vi "Result.Test Result to CSV.vi"(6 "SummaryOnly":bool, 7 "Exclude Header CSV":bool, 8 "error in":errorcluster, 9 "Test Result":T1={"#attributes"={"Version"="MTE_1.0.0"}, "Station"={"Name"="", "PN"="", "SN"="", "Rev"="", "PC Name"="", "Location"="", "HW_Config"={"HW_Item"=[]}, "SW_Config"={"SW_Item"=[]}}, "Test Run"={"Operator"="", "Start Time"=timestamp(0 s since 1904-01-01), "Duration(s)"=0.0, "Mode"="", "Comment"="", "ProcessStep"=""}, "Test Sequence"={"Name"="", "Config"={"Config_Item"=[]}}, "UUTs"={"UUT"=[]}} {"UUTs"."UUT"."Measurements"."Measurement"."Status" items=["LOG", "PASS", "FAIL", "ERROR"]}, 10 "File Name":string, 11 "Dir":path) -> (0 "error out":errorcluster, 3 "File Out":path)   [LabVIEW 2018]
uses:
  Result XML/TestResult.FullResultData.ctl
  Result XML/TestResult.Station Info.ctl
  Result XML/TestResult.HW Item.ctl
  Result XML/TestResult.SW Item.ctl
  Result XML/TestResult.Test Run Info.ctl
  Result XML/TestResult.Test Info.ctl
  Result XML/TestResult.UUT Result.ctl
  Result XML/TestResult.Symptom.ctl
  Result XML/TestResult.Symptom.State.ctl
  Result.Measurement Item.ctl
  Result.Measurement and Attribute Item Status.ctl
  Result XML/TestResult.UUTInfo.ctl
  <vilib>/KATE/Files/File Utils.lvlib
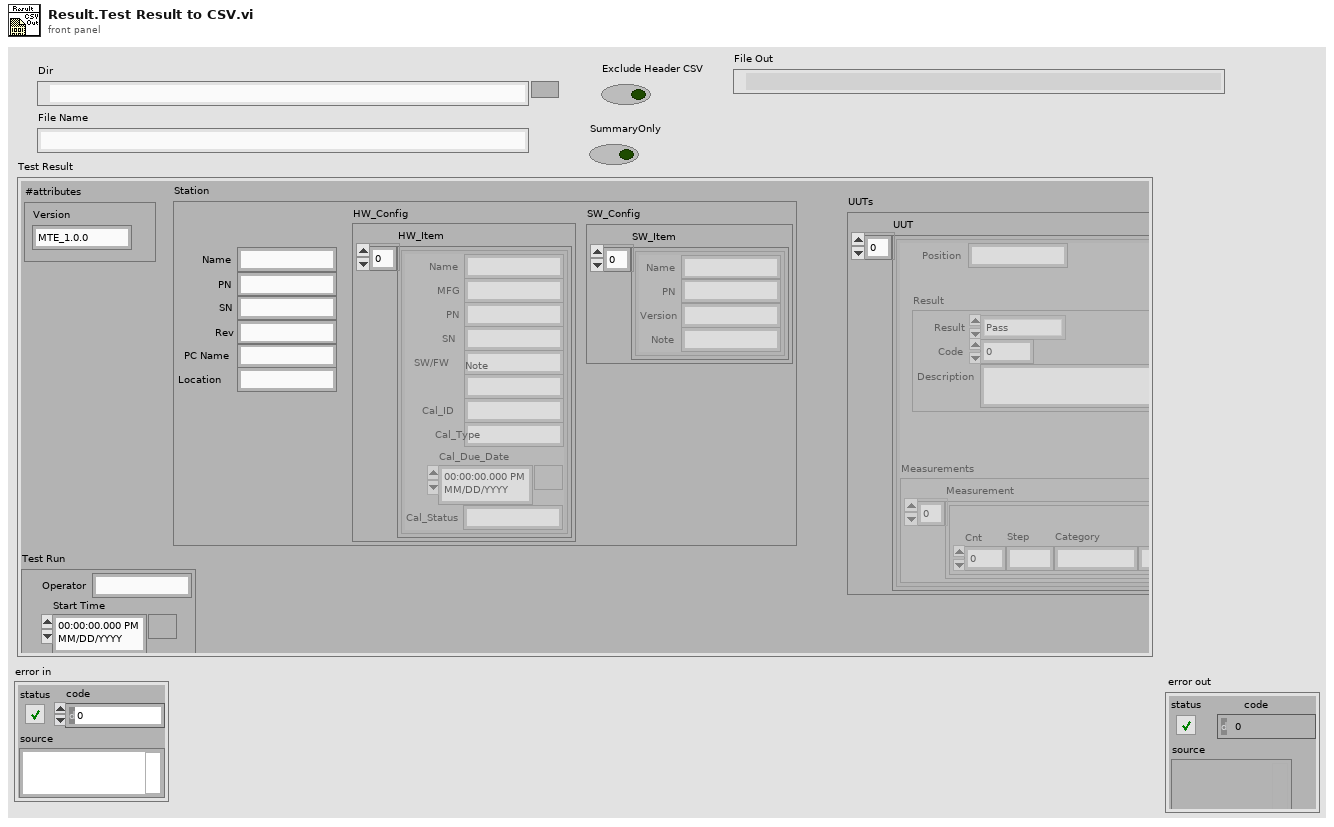
[diagram p1: front panel]
types:
  T1 = typedef "TestResult.FullResultData.ctl" = cluster{"#attributes":cluster{"Version":string}, "Station":T2, "Test Run":T5, "Test Sequence":T6, "UUTs":cluster{"UUT":T7[]}}
  T2 = typedef "TestResult.Station Info.ctl" = cluster{"Name":string, "PN":string, "SN":string, "Rev":string, "PC Name":string, "Location":string, "HW_Config":cluster{"HW_Item":T3[]}, "SW_Config":cluster{"SW_Item":T4[]}}
  T3 = typedef "TestResult.HW Item.ctl" = cluster{"Name":string, "MFG":string, "PN":string, "SN":string, "SW/FW":string, "Note":string, "Cal_ID":string, "Cal_Type":string, "Cal_Due_Date":timestamp, "Cal_Status":string}
  T4 = typedef "TestResult.SW Item.ctl" = cluster{"Name":string, "PN":string, "Version":string, "Note":string}
  T5 = typedef "TestResult.Test Run Info.ctl" = cluster{"Operator":string, "Start Time":timestamp, "Duration(s)":dbl, "Mode":string, "Comment":string, "ProcessStep":string}
  T6 = typedef "TestResult.Test Info.ctl" = cluster{"Name":string, "Config":cluster{"Config_Item":cluster{"Name":string, "Value":string}[]}}
  T7 = typedef "TestResult.UUT Result.ctl" = cluster{"Position":string, "Result":T8, "Measurements":cluster{"Measurement":T10[]}, "UUTInfo":T12}
  T8 = typedef "TestResult.Symptom.ctl" = cluster{"Result":T9, "Code":i32, "Description":string}
  T9 = typedef "TestResult.Symptom.State.ctl" = enum16{"Pass", "Fail", "Error", "Aborted", "Completed", "Logged"}
  T10 = typedef "Result.Measurement Item.ctl" = cluster{"Cnt":i32, "Step":string, "Category":string, "Name":string, "Value":string, "Units":string, "LimType":string, "LL":string, "UL":string, "Status":T11, "Code":i32, "Desc":string, "Time":timestamp}
  T11 = typedef "Result.Measurement and Attribute Item Status.ctl" = i32
  T12 = typedef "TestResult.UUTInfo.ctl" = cluster{"Product":string, "Desc":string, "PN":string, "SN":string, "Lot":string, "DateCode":string, "AltID":string, "Revision":string, "Properties":cluster{"Property":cluster{"Name":string, "Value":string}[]}}
  T13 = enum16{"open", "replace", "create", "open or create", "replace or create", "replace or create with confirmation"}
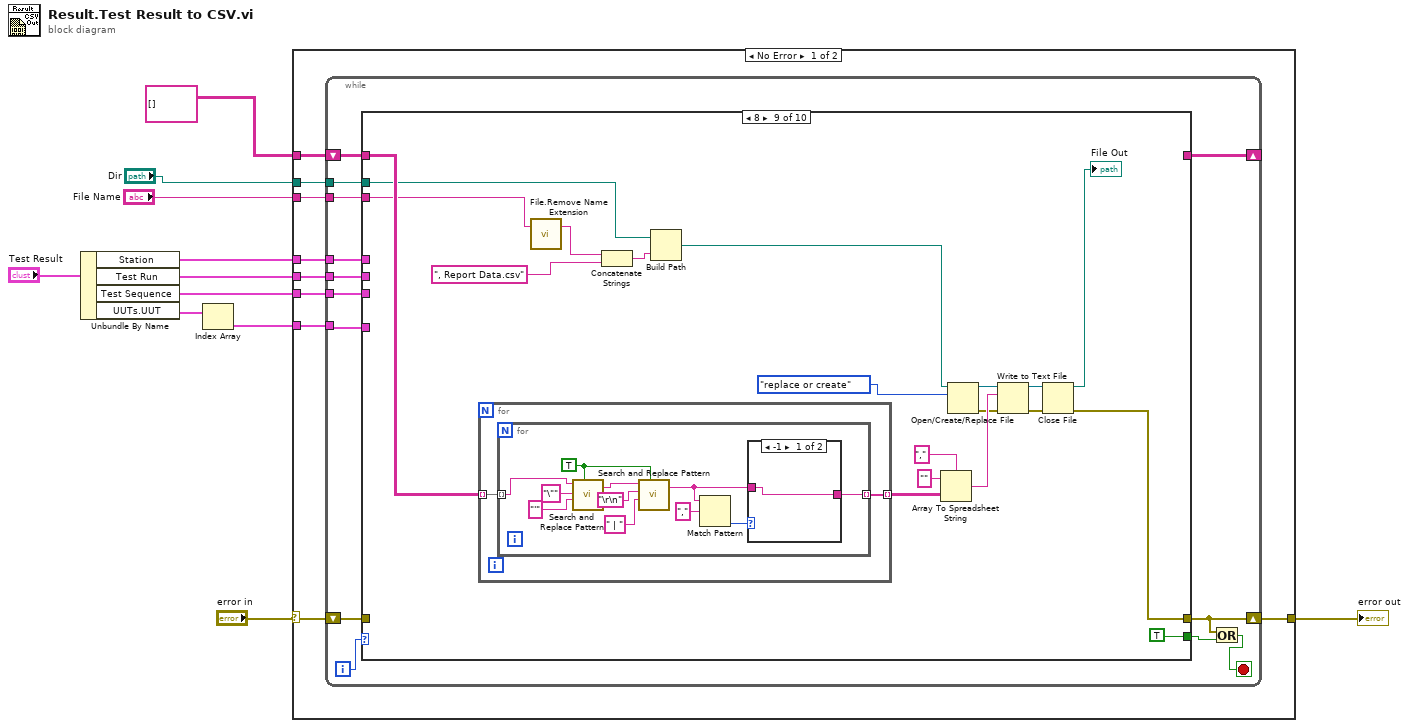
[diagram p0: block diagram]
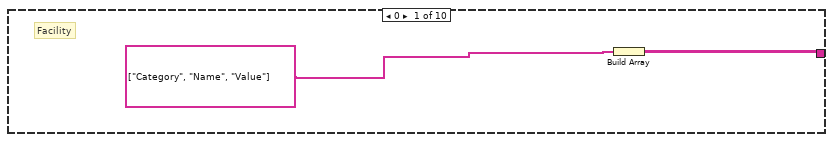
[diagram p2: hidden frame]
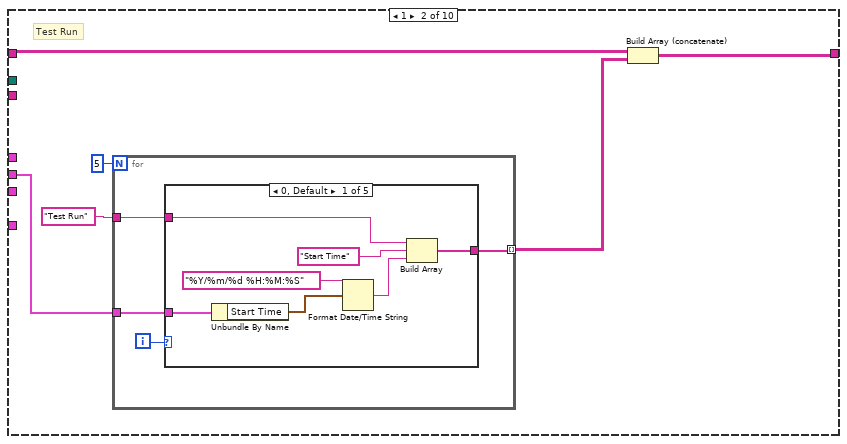
[diagram p3: hidden frame]
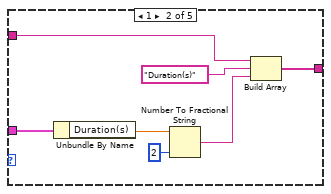
[diagram p4: hidden frame]
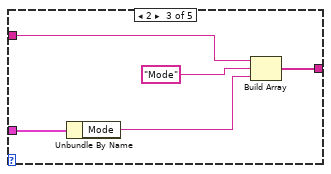
[diagram p5: hidden frame]
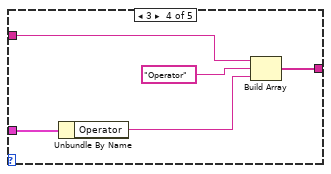
[diagram p6: hidden frame]
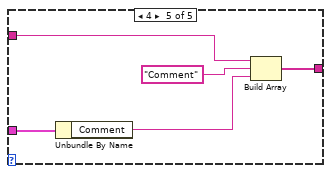
[diagram p7: hidden frame]
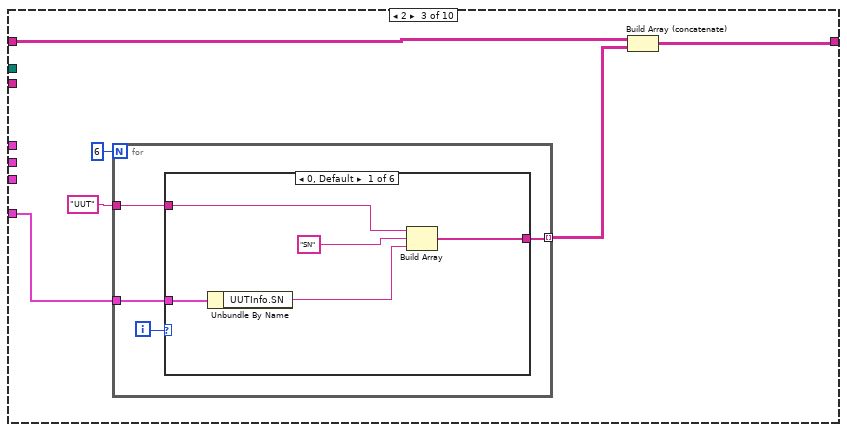
[diagram p8: hidden frame]
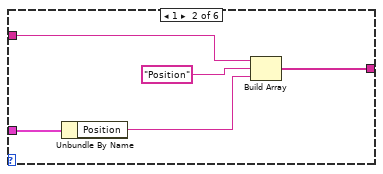
[diagram p9: hidden frame]
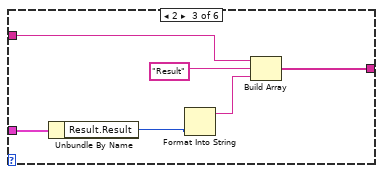
[diagram p10: hidden frame]
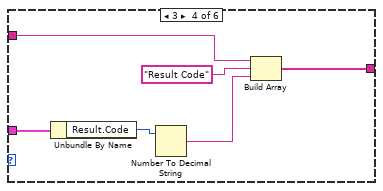
[diagram p11: hidden frame]
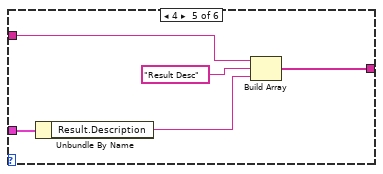
[diagram p12: hidden frame]
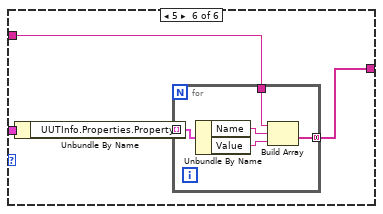
[diagram p13: hidden frame]
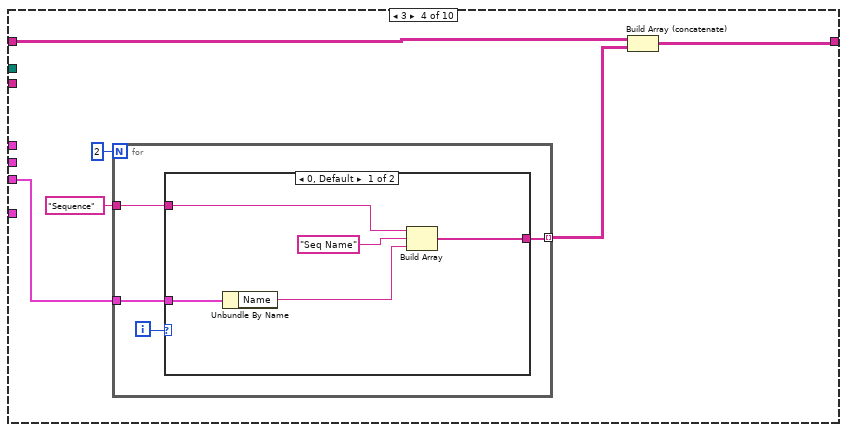
[diagram p14: hidden frame]
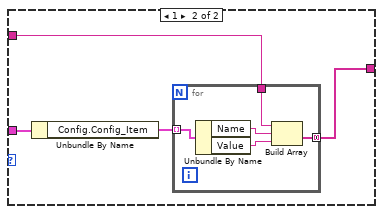
[diagram p15: hidden frame]
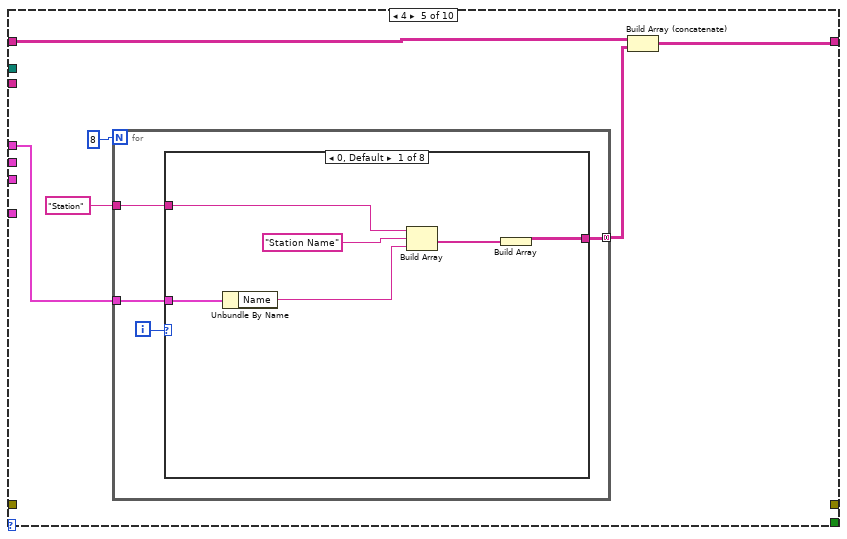
[diagram p16: hidden frame]
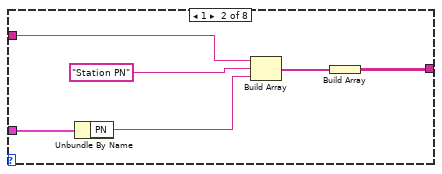
[diagram p17: hidden frame]
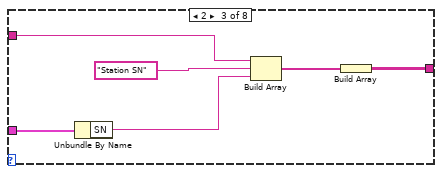
[diagram p18: hidden frame]
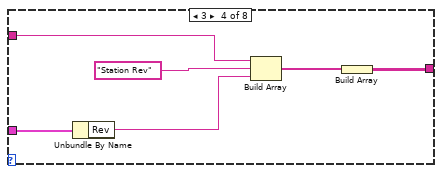
[diagram p19: hidden frame]
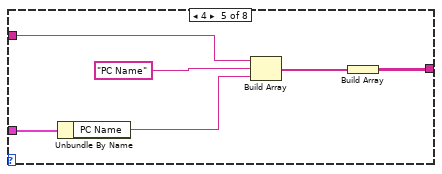
[diagram p20: hidden frame]
diagram:
  n1 = Unbundle By Name("Test Result") -> ("Station"=w6:T2, "Test Run"=w5:T5, "Test Sequence"=w4:T6, "UUTs.UUT"=w8:T7[])
  n2 = Index Array(array=w8) -> (element=w7:T7)  [unwired: 1 in]
  n3 = case shown="No Error" "error in" {
    selector: "error in" -> [w19 w492]
    tunnel: [w20 w492] -> w11
    tunnel: w7 -> [w18 _]
    tunnel: w6 -> [w17 _]
    tunnel: w5 -> [w16 _]
    tunnel: w4 -> [w15 _]
    tunnel: "File Name" -> [w14 _]
    tunnel: "Dir" -> [w13 _]
    tunnel: string[][] [] -> [w12 _]
    frame No Error {
      n4 = while {
        shift-right: [w23] -> w20
        shift-left: w19 -> [w33]
        shift-right: [w26] -> _
        shift-left: w12 -> [w32]
        tunnel: w18 -> [w29]
        tunnel: w17 -> [w28]
        tunnel: w16 -> [w30]
        tunnel: w15 -> [w27]
        tunnel: w14 -> [w25]
        tunnel: w13 -> [w24]
        i -> [w31]
        stop <- w21 stop-if-true
        n5 = case shown="8" w31 {
          tunnel: [_ _ _ _ _ w216 _ _ w455 w490] -> w23
          tunnel: w33 -> [_ _ _ _ _ _ _ _ _ w490]
          tunnel: w32 -> [_ w36 w77 w123 w148 w217 _ w429 w462 _]
          tunnel: [w35 w37 w75 w121 w145 _ w260 w430 _ _] -> w26
          tunnel: w30 -> [_ w38 _ _ _ _ w255 _ _ _]
          tunnel: w29 -> [_ _ w76 _ _ _ w258 w432 _ _]
          tunnel: w28 -> [_ _ _ _ w147 _ w254 _ _ _]
          tunnel: w27 -> [_ _ _ w122 _ _ w253 _ _ _]
          tunnel: [_ _ _ _ _ "SummaryOnly" _ _ TRUE TRUE] -> w22
          tunnel: w25 -> [_ _ _ _ _ w227 _ _ w458 _]
          tunnel: w24 -> [_ _ _ _ _ w224 _ _ w457 _]
          frame 0 {
            # "Facility"
            n6 = Build Array(string[] ["Category", "Name", "Value"]) -> (w35:string[][])
          }
          frame 1 {
            # "Test Run"
            n7 = for {
              N: 5 -> [_]
              tunnel: w38 -> [w45]
              tunnel: [w43] -> w39 mode=indexing
              tunnel: "Test Run" -> [w42]
              i -> [w44]
              n8 = case shown="0, Default" w44 {
                tunnel: w45 -> [w51 w59 w64 w69 w74]
                tunnel: [w47 w57 w62 w67 w72] -> w43
                tunnel: w42 -> [w46 w56 w61 w66 w71]
                frame 0, Default {
                  n9 = Unbundle By Name(w51) -> ("Start Time"=w48:timestamp)
                  n10 = Format Date/Time String(time format string (%c)="%Y/%m/%d %H:%M:%S", seconds (now)=w48) -> (date/time string=w49:string)  [unwired: 1 in]
                  n11 = Build Array(w46, "Start Time", w49) -> (w47:string[])
                }
                frame 1 {
                  n12 = Unbundle By Name(w59) -> ("Duration(s)"=w55:dbl)
                  n13 = Number To Fractional String(number=w55, precision (6)=i16 2) -> (F-format string=w53:string)  [unwired: 2 in]
                  n14 = Build Array(w56, "Duration(s)", w53) -> (w57:string[])
                }
                frame 2 {
                  n15 = Unbundle By Name(w64) -> ("Mode"=w60:string)
                  n16 = Build Array(w61, "Mode", w60) -> (w62:string[])
                }
                frame 3 {
                  n17 = Unbundle By Name(w69) -> ("Operator"=w65:string)
                  n18 = Build Array(w66, "Operator", w65) -> (w67:string[])
                }
                frame 4 {
                  n19 = Unbundle By Name(w74) -> ("Comment"=w70:string)
                  n20 = Build Array(w71, "Comment", w70) -> (w72:string[])
                }
              }
            }
            n21 = Build Array (concatenate)(w36, w39) -> (w37:string[][])
          }
          frame 2 {
            n22 = for {
              N: 6 -> [_]
              tunnel: w76 -> [w84]
              tunnel: [w82] -> w78 mode=indexing
              tunnel: "UUT" -> [w81]
              i -> [w83]
              n23 = case shown="0, Default" w83 {
                tunnel: w84 -> [w89 w94 w100 w106 w111 w115]
                tunnel: [w87 w92 w99 w104 w109 w112] -> w82
                tunnel: w81 -> [w86 w91 w98 w103 w108 w113]
                frame 0, Default {
                  n24 = Unbundle By Name(w89) -> ("UUTInfo.SN"=w85:string)
                  n25 = Build Array(w86, "SN", w85) -> (w87:string[])
                }
                frame 1 {
                  n26 = Unbundle By Name(w94) -> ("Position"=w90:string)
                  n27 = Build Array(w91, "Position", w90) -> (w92:string[])
                }
                frame 2 {
                  n28 = Unbundle By Name(w100) -> ("Result.Result"=w96:T9)
                  n29 = Format Into String(w96) -> (resulting string=w95:string)  [unwired: 3 in, 1 out]
                  n30 = Build Array(w98, "Result", w95) -> (w99:string[])
                }
                frame 3 {
                  n31 = Unbundle By Name(w106) -> ("Result.Code"=w102:i32)
                  n32 = Number To Decimal String(number=w102) -> (decimal integer string=w101:string)  [unwired: 1 in]
                  n33 = Build Array(w103, "Result Code", w101) -> (w104:string[])
                }
                frame 4 {
                  n34 = Unbundle By Name(w111) -> ("Result.Description"=w107:string)
                  n35 = Build Array(w108, "Result Desc", w107) -> (w109:string[])
                }
                frame 5 {
                  n36 = Unbundle By Name(w115) -> ("UUTInfo.Properties.Property"=w114:cluster{"Name":string, "Value":string}[])
                  n37 = for {
                    tunnel: w114 -> [w120] mode=indexing
                    tunnel: [w117] -> w112 mode=concatenating
                    tunnel: w113 -> [w116]
                    n38 = Unbundle By Name(w120) -> ("Name"=w119:string, "Value"=w118:string)
                    n39 = Build Array(w116, w119, w118) -> (w117:string[])
                  }
                }
              }
            }
            n40 = Build Array (concatenate)(w77, w78) -> (w75:string[][])
          }
          frame 3 {
            n41 = for {
              N: 2 -> [_]
              tunnel: w122 -> [w130]
              tunnel: [w128] -> w124 mode=indexing
              tunnel: "Sequence" -> [w127]
              i -> [w129]
              n42 = case shown="0, Default" w129 {
                tunnel: w130 -> [w135 w139]
                tunnel: [w133 w136] -> w128
                tunnel: w127 -> [w132 w137]
                frame 0, Default {
                  n43 = Unbundle By Name(w135) -> ("Name"=w131:string)
                  n44 = Build Array(w132, "Seq Name", w131) -> (w133:string[])
                }
                frame 1 {
                  n45 = Unbundle By Name(w139) -> ("Config.Config_Item"=w138:cluster{"Name":string, "Value":string}[])
                  n46 = for {
                    tunnel: w138 -> [w144] mode=indexing
                    tunnel: [w141] -> w136 mode=concatenating
                    tunnel: w137 -> [w140]
                    n47 = Unbundle By Name(w144) -> ("Name"=w143:string, "Value"=w142:string)
                    n48 = Build Array(w140, w143, w142) -> (w141:string[])
                  }
                }
              }
            }
            n49 = Build Array (concatenate)(w123, w124) -> (w121:string[][])
          }
          frame 4 {
            n50 = for {
              N: 8 -> [_]
              tunnel: w147 -> [w154]
              tunnel: [w152] -> w146 mode=concatenating
              tunnel: "Station" -> [w151]
              i -> [w153]
              n51 = case shown="0, Default" w153 {
                tunnel: w154 -> [w160 w166 w172 w178 w184 w190 w196 w205]
                tunnel: [w155 w161 w167 w173 w179 w185 w193 w202] -> w152
                tunnel: w151 -> [w158 w164 w171 w177 w183 w189 _ _]
                frame 0, Default {
                  n52 = Unbundle By Name(w160) -> ("Name"=w157:string)
                  n53 = Build Array(w158, "Station Name", w157) -> (w156:string[])
                  n54 = Build Array(w156) -> (w155:string[][])
                }
                frame 1 {
                  n55 = Unbundle By Name(w166) -> ("PN"=w163:string)
                  n56 = Build Array(w164, "Station PN", w163) -> (w162:string[])
                  n57 = Build Array(w162) -> (w161:string[][])
                }
                frame 2 {
                  n58 = Unbundle By Name(w172) -> ("SN"=w169:string)
                  n59 = Build Array(w171, "Station SN", w169) -> (w168:string[])
                  n60 = Build Array(w168) -> (w167:string[][])
                }
                frame 3 {
                  n61 = Unbundle By Name(w178) -> ("Rev"=w175:string)
                  n62 = Build Array(w177, "Station Rev", w175) -> (w174:string[])
                  n63 = Build Array(w174) -> (w173:string[][])
                }
                frame 4 {
                  n64 = Unbundle By Name(w184) -> ("PC Name"=w181:string)
                  n65 = Build Array(w183, "PC Name", w181) -> (w180:string[])
                  n66 = Build Array(w180) -> (w179:string[][])
                }
                frame 5 {
                  n67 = Unbundle By Name(w190) -> ("Location"=w187:string)
                  n68 = Build Array(w189, "Station Location", w187) -> (w186:string[])
                  n69 = Build Array(w186) -> (w185:string[][])
                }
                frame 6 {
                  n70 = Unbundle By Name(w196) -> ("HW_Config.HW_Item"=w195:T3[])
                  n71 = for {
                    tunnel: w195 -> [w197] mode=indexing
                    tunnel: [w198] -> w192 mode=indexing
                    tunnel: "Equipment List" -> [w199]
                    n72 = call "Result.Equipment List Item to 1D Array.vi"("Eq Item"=w197, "Category"=w199) -> ("List"=w198:string[])  [unwired: 9 in]
                  }
                  n73 = Build Array (concatenate)(string[] ["Category", "Name", "PN", "SN", "SW/FW", "Cal ID", "Cal Type", "Cal Due", "Cal Status"], w192) -> (w193:string[][])
                }
                frame 7 {
                  n74 = Unbundle By Name(w205) -> ("SW_Config.SW_Item"=w204:T4[])
                  n75 = for {
                    tunnel: w204 -> [w212] mode=indexing
                    tunnel: [w206] -> w201 mode=indexing
                    tunnel: "SW List" -> [w207]
                    n76 = Unbundle By Name(w212) -> ("Name"=w208:string, "PN"=w209:string, "Version"=w210:string, "Note"=w211:string)
                    n77 = Build Array(w207, w208, w209, w210, w211) -> (w206:string[])
                  }
                  n78 = Build Array (concatenate)(string[] ["Category", "Name", "PN", "Version", "Note"], w201) -> (w202:string[][])
                }
              }
            }
            n79 = Build Array (concatenate)(w148, w146) -> (w145:string[][])
          }
          frame 5 {
            n80 = for {
              tunnel: w217 -> [w237] mode=indexing
              tunnel: [w236] -> w222 mode=indexing
              n81 = for {
                tunnel: w237 -> [w245] mode=indexing
                tunnel: [w248] -> w236 mode=indexing
                w243 = TRUE ("replace all? (F)")
                n82 = call <vilib>:"Search and Replace Pattern.vi"("string"=w245, "regular expression (\"\")"="\"", "replace string (\"\")"="'", "replace all? (F)"=w243) -> ("result string"=w244:string)  [unwired: 1 in, 1 out]
                n83 = call <vilib>:"Search and Replace Pattern.vi"("string"=w244, "regular expression (\"\")"="\n", "replace string (\"\")"=" | ", "replace all? (F)"=w243) -> ("result string"=w240:string)  [unwired: 1 in, 1 out]
                n84 = Match Pattern(string=w240, regular expression=",") -> (offset past match=w238:i32)  [unwired: 1 in, 3 out]
                n85 = case shown="-1" w238 {
                  tunnel: [w249 w251] -> w248
                  tunnel: w240 -> [w249 w250]
                  frame -1 {
                  }
                  frame 0, Default {
                    w252 = "\""
                    n86 = Concatenate Strings(w252, w250, w252) -> (w251:string)
                  }
                }
              }
            }
            n87 = call <vilib>:"File.Remove Name Extension.vi"("File Name"=w227) -> ("Name Less Ext"=w215:string)  [unwired: 1 in, 1 out]
            n88 = Concatenate Strings(w215, ", Report Header.csv" ("string")) -> (w225:string)
            n89 = Build Path(base path=w224, name or relative path=w225) -> (appended path=w218:path)
            n90 = Array To Spreadsheet String(delimiter (Tab)=",", array=w222, 3:"" ("format string")) -> (spreadsheet string=w223:string)
            n91 = case shown="False" "Exclude Header CSV" {
              tunnel: w223 -> [w235 _]
              tunnel: T13."replace or create" ("operation (0:open)") -> [w230 _]
              tunnel: w218 -> [w229 _]
              tunnel: [w228 _] -> w216
              frame False {
                n92 = Open/Create/Replace File(file path (use dialog)=w229, operation (0:open)=w230) -> (refnum out=w232:refnum<file>, error out=w233:errorcluster)  [unwired: 4 in, 1 out]
                n93 = Write to Text File(file (use dialog)=w232, text=w235, error in=w233) -> (refnum out=w231:refnum<file>, error out=w234:errorcluster)  [unwired: 1 in, 1 out]
                n94 = Close File(refnum=w231, error in=w234) -> (error out=w228:errorcluster)  [unwired: 1 out]
              }
              frame True {
              }
            }
          }
          frame 6 {
            # "SN\nPosition\nTime\nMode\nComment\nResult\nCode\nDesc\nDur\nOper"
            n95 = while {
              tunnel: w258 -> [w269]
              tunnel: [w267] -> w257 mode=indexing if=w263
              tunnel: string[] ["0", "0", "Header"] -> [w266]
              tunnel: w255 -> [w265]
              tunnel: w254 -> [w264]
              tunnel: w253 -> [w262]
              i -> [w268]
              stop <- w261 stop-if-true
              n96 = case shown="1" w268 {
                tunnel: w269 -> [w270 w275 _ _ _ _ w305 w311 w316 _ _ _ _ _ _ _ _ _ _ _ _ _ _]
                tunnel: [w273 w278 w282 w290 w295 w300 w307 w313 w318 w324 w329 w334 w344 w353 w362 w371 w380 w389 w398 w407 w416 w425 w427] -> w267
                tunnel: w266 -> [w271 w276 w280 w288 w293 w298 w306 w312 w317 w320 w327 w332 _ _ _ _ _ _ _ _ _ _ w427]
                tunnel: w265 -> [_ _ w281 w287 _ w297 _ _ _ w319 w326 _ _ _ _ _ _ _ _ _ _ _ _]
                tunnel: w264 -> [_ _ _ _ _ _ _ _ _ _ _ w331 w343 w352 w361 w370 w379 w388 w397 w406 w415 w424 _]
                tunnel: [_ _ _ _ _ _ _ _ _ _ _ _ w336 w345 w354 w363 w372 w381 w390 w399 w408 w417 TRUE] -> w261
                tunnel: w262 -> [_ _ _ _ w292 _ _ _ _ _ _ _ _ _ _ _ _ _ _ _ _ _ _]
                frame 0 {
                  n97 = Unbundle By Name(w270) -> ("UUTInfo.SN"=w272:string)
                  n98 = Build Array (concatenate)(w271, "SN", w272) -> (w273:string[])
                }
                frame 1 {
                  n99 = Unbundle By Name(w275) -> ("Position"=w277:string)
                  n100 = Build Array (concatenate)(w276, "Position", w277) -> (w278:string[])
                }
                frame 2 {
                  n101 = Unbundle By Name(w281) -> ("Start Time"=w283:timestamp)
                  n102 = Format Date/Time String(time format string (%c)="%Y/%m/%d %H:%M:%S", seconds (now)=w283) -> (date/time string=w284:string)  [unwired: 1 in]
                  n103 = Build Array (concatenate)(w280, "Start Time", w284) -> (w282:string[])
                }
                frame 3 {
                  n104 = Unbundle By Name(w287) -> ("Mode"=w289:string)
                  n105 = Build Array (concatenate)(w288, "Mode", w289) -> (w290:string[])
                }
                frame 4 {
                  n106 = Unbundle By Name(w292) -> ("Name"=w294:string)
                  n107 = Build Array (concatenate)(w293, "Sequence", w294) -> (w295:string[])
                }
                frame 5 {
                  n108 = Unbundle By Name(w297) -> ("Comment"=w299:string)
                  n109 = Build Array (concatenate)(w298, "Comment", w299) -> (w300:string[])
                }
                frame 6 {
                  n110 = Unbundle By Name(w305) -> ("Result.Result"=w303:T9)
                  n111 = Format Into String(w303) -> (resulting string=w302:string)  [unwired: 3 in, 1 out]
                  n112 = Build Array (concatenate)(w306, "Result", w302) -> (w307:string[])
                }
                frame 7 {
                  n113 = Unbundle By Name(w311) -> ("Result.Code"=w309:i32)
                  n114 = Format Into String(w309) -> (resulting string=w308:string)  [unwired: 3 in, 1 out]
                  n115 = Build Array (concatenate)(w312, "Result Code", w308) -> (w313:string[])
                }
                frame 8 {
                  n116 = Unbundle By Name(w316) -> ("Result.Description"=w314:string)
                  n117 = Build Array (concatenate)(w317, "Result Desc", w314) -> (w318:string[])
                }
                frame 9 {
                  n118 = Unbundle By Name(w319) -> ("Duration(s)"=w323:dbl)
                  n119 = Number To Fractional String(number=w323, precision (6)=i16 2) -> (F-format string=w321:string)  [unwired: 2 in]
                  n120 = Build Array (concatenate)(w320, "Duration(s)", w321) -> (w324:string[])
                }
                frame 10 {
                  n121 = Unbundle By Name(w326) -> ("Operator"=w328:string)
                  n122 = Build Array (concatenate)(w327, "Operator", w328) -> (w329:string[])
                }
                frame 11 {
                  n123 = Unbundle By Name(w331) -> ("Location"=w333:string)
                  n124 = Build Array (concatenate)(w332, "Location", w333) -> (w334:string[])
                }
                frame 12 {
                  n125 = Unbundle By Name(w343) -> ("SW_Config.SW_Item"=w342:T4[])
                  n126 = Index Array(array=w342, index=0) -> (element=w341:T4)
                  n127 = Unbundle By Name(w341) -> ("Name"=w339:string, "Version"=w340:string)
                  n128 = Build Array (concatenate)(string[] ["0", "0", "SW"], w339, w340) -> (w344:string[])
                  n129 = Empty String/Path?(string/path=w339) -> (empty?=w336:bool)
                }
                frame 13 {
                  n130 = Unbundle By Name(w352) -> ("SW_Config.SW_Item"=w351:T4[])
                  n131 = Index Array(array=w351, index=1) -> (element=w350:T4)
                  n132 = Unbundle By Name(w350) -> ("Name"=w348:string, "Version"=w349:string)
                  n133 = Build Array (concatenate)(string[] ["0", "0", "SW"], w348, w349) -> (w353:string[])
                  n134 = Empty String/Path?(string/path=w348) -> (empty?=w345:bool)
                }
                frame 14 {
                  n135 = Unbundle By Name(w361) -> ("SW_Config.SW_Item"=w360:T4[])
                  n136 = Index Array(array=w360, index=2) -> (element=w359:T4)
                  n137 = Unbundle By Name(w359) -> ("Name"=w357:string, "Version"=w358:string)
                  n138 = Build Array (concatenate)(string[] ["0", "0", "SW"], w357, w358) -> (w362:string[])
                  n139 = Empty String/Path?(string/path=w357) -> (empty?=w354:bool)
                }
                frame 15 {
                  n140 = Unbundle By Name(w370) -> ("SW_Config.SW_Item"=w369:T4[])
                  n141 = Index Array(array=w369, index=3) -> (element=w368:T4)
                  n142 = Unbundle By Name(w368) -> ("Name"=w366:string, "Version"=w367:string)
                  n143 = Build Array (concatenate)(string[] ["0", "0", "SW"], w366, w367) -> (w371:string[])
                  n144 = Empty String/Path?(string/path=w366) -> (empty?=w363:bool)
                }
                frame 16 {
                  n145 = Unbundle By Name(w379) -> ("SW_Config.SW_Item"=w378:T4[])
                  n146 = Index Array(array=w378, index=4) -> (element=w377:T4)
                  n147 = Unbundle By Name(w377) -> ("Name"=w375:string, "Version"=w376:string)
                  n148 = Build Array (concatenate)(string[] ["0", "0", "SW"], w375, w376) -> (w380:string[])
                  n149 = Empty String/Path?(string/path=w375) -> (empty?=w372:bool)
                }
                frame 17 {
                  n150 = Unbundle By Name(w388) -> ("SW_Config.SW_Item"=w387:T4[])
                  n151 = Index Array(array=w387, index=5) -> (element=w386:T4)
                  n152 = Unbundle By Name(w386) -> ("Name"=w384:string, "Version"=w385:string)
                  n153 = Build Array (concatenate)(string[] ["0", "0", "SW"], w384, w385) -> (w389:string[])
                  n154 = Empty String/Path?(string/path=w384) -> (empty?=w381:bool)
                }
                frame 18 {
                  n155 = Unbundle By Name(w397) -> ("SW_Config.SW_Item"=w396:T4[])
                  n156 = Index Array(array=w396, index=6) -> (element=w395:T4)
                  n157 = Unbundle By Name(w395) -> ("Name"=w393:string, "Version"=w394:string)
                  n158 = Build Array (concatenate)(string[] ["0", "0", "SW"], w393, w394) -> (w398:string[])
                  n159 = Empty String/Path?(string/path=w393) -> (empty?=w390:bool)
                }
                frame 19 {
                  n160 = Unbundle By Name(w406) -> ("SW_Config.SW_Item"=w405:T4[])
                  n161 = Index Array(array=w405, index=7) -> (element=w404:T4)
                  n162 = Unbundle By Name(w404) -> ("Name"=w402:string, "Version"=w403:string)
                  n163 = Build Array (concatenate)(string[] ["0", "0", "SW"], w402, w403) -> (w407:string[])
                  n164 = Empty String/Path?(string/path=w402) -> (empty?=w399:bool)
                }
                frame 20 {
                  n165 = Unbundle By Name(w415) -> ("SW_Config.SW_Item"=w414:T4[])
                  n166 = Index Array(array=w414, index=8) -> (element=w413:T4)
                  n167 = Unbundle By Name(w413) -> ("Name"=w411:string, "Version"=w412:string)
                  n168 = Build Array (concatenate)(string[] ["0", "0", "SW"], w411, w412) -> (w416:string[])
                  n169 = Empty String/Path?(string/path=w411) -> (empty?=w408:bool)
                }
                frame 21 {
                  n170 = Unbundle By Name(w424) -> ("SW_Config.SW_Item"=w423:T4[])
                  n171 = Index Array(array=w423, index=9) -> (element=w422:T4)
                  n172 = Unbundle By Name(w422) -> ("Name"=w420:string, "Version"=w421:string)
                  n173 = Build Array (concatenate)(string[] ["0", "0", "SW"], w420, w421) -> (w425:string[])
                  n174 = Empty String/Path?(string/path=w420) -> (empty?=w417:bool)
                }
                frame Default {
                }
              }
              n175 = Not(x=w261) -> (.not. x?=w263:bool)
            }
            n176 = Build Array (concatenate)(string[] ["Order", "Step", "Category", "Name", "Value", "Units", "LimType", "LL", "UL", "Result", "Result Code", "Result Desc"], w257) -> (w260:string[][])
          }
          frame 7 {
            (unwired) string[] ["Order", "Step", "Category", "Name", "Value", "Units", "LimType", "LL", "UL", "Result", "Result Code", "Result Desc"]
            n177 = Unbundle By Name(w432) -> ("Measurements.Measurement"=w428:T10[])
            n178 = for {
              tunnel: w428 -> [w449] mode=indexing
              tunnel: [w435] -> w431 mode=indexing
              n179 = Unbundle By Name(w449) -> ("Cnt"=w448:i32, "Step"=w446:string, "Category"=w445:string, "Name"=w444:string, "Value"=w443:string, "Units"=w442:string, "LimType"=w441:string, "LL"=w440:string, "UL"=w439:string, "Status"=w434:T11, "Code"=w438:i32, "Desc"=w436:string)
              n180 = case shown="3" w434 {
                tunnel: ["LOG" "PASS" "FAIL" "ERROR"] -> w433
                frame 0, Default {
                }
                frame 1 {
                }
                frame 2 {
                }
                frame 3 {
                }
              }
              n181 = Number To Decimal String(number=w448) -> (decimal integer string=w447:string)  [unwired: 1 in]
              n182 = Number To Decimal String(number=w438) -> (decimal integer string=w437:string)  [unwired: 1 in]
              n183 = Build Array(w447, w446, w445, w444, w443, w442, w441, w440, w439, w433, w437, w436) -> (w435:string[])
            }
            n184 = Build Array (concatenate)(w429, w431) -> (w430:string[][])
          }
          frame 8 {
            n185 = for {
              tunnel: w462 -> [w474] mode=indexing
              tunnel: [w473] -> w466 mode=indexing
              n186 = for {
                tunnel: w474 -> [w482] mode=indexing
                tunnel: [w485] -> w473 mode=indexing
                w480 = TRUE ("replace all? (F)")
                n187 = call <vilib>:"Search and Replace Pattern.vi"("string"=w482, "regular expression (\"\")"="\"", "replace string (\"\")"="'", "replace all? (F)"=w480) -> ("result string"=w481:string)  [unwired: 1 in, 1 out]
                n188 = call <vilib>:"Search and Replace Pattern.vi"("string"=w481, "regular expression (\"\")"="\r\n", "replace string (\"\")"=" | ", "replace all? (F)"=w480) -> ("result string"=w477:string)  [unwired: 1 in, 1 out]
                n189 = Match Pattern(string=w477, regular expression=",") -> (offset past match=w475:i32)  [unwired: 1 in, 3 out]
                n190 = case shown="-1" w475 {
                  tunnel: [w486 w488] -> w485
                  tunnel: w477 -> [w486 w487]
                  frame -1 {
                  }
                  frame 0, Default {
                    w489 = "\""
                    n191 = Concatenate Strings(w489, w487, w489) -> (w488:string)
                  }
                }
              }
            }
            n192 = call <vilib>:"File.Remove Name Extension.vi"("File Name"=w458) -> ("Name Less Ext"=w461:string)  [unwired: 1 in, 1 out]
            n193 = Concatenate Strings(w461, ", Report Data.csv" ("string")) -> (w459:string)
            n194 = Build Path(base path=w457, name or relative path=w459) -> (appended path=w456:path)
            n195 = Array To Spreadsheet String(delimiter (Tab)=",", array=w466, 3:"" ("format string")) -> (spreadsheet string=w471:string)
            n196 = Open/Create/Replace File(file path (use dialog)=w456, operation (0:open)=T13."replace or create") -> (refnum out=w468:refnum<file>, error out=w469:errorcluster)  [unwired: 4 in, 1 out]
            n197 = Write to Text File(file (use dialog)=w468, text=w471, error in=w469) -> (refnum out=w467:refnum<file>, error out=w470:errorcluster)  [unwired: 1 in, 1 out]
            n198 = Close File(refnum=w467, error in=w470) -> (path=→"File Out":path, error out=w455:errorcluster)
          }
          frame Default {
          }
        }
        n199 = Or(x=w23, y=w22) -> (x .or. y?=w21:bool)
      }
    }
    frame Error {
    }
  }
  "error out" <- w11
